vi "Waveform and Laser Controls V3.vi"() -> ()   [LabVIEW 2014]
uses:
  Waveform Scan Parameters.ctl
  <vilib>/Platform/TimedLoop/XDataNode/timing_clust.ctl
  <vilib>/Platform/TimedLoop/XDataNode/nitl_modes.ctl
  <vilib>/Platform/TimedLoop/XDataNode/wakeup.ctl
  <vilib>/rvi/Emulation/niFpgaGetClockAttributes.vi
  <vilib>/rvi/Emulation/niFpgaSctlEmulationGetInTimedLoop.vi
  <vilib>/rvi/Emulation/niFpgaEmulationReportErrorSimple.vi
  <vilib>/rvi/eio/common/nirviEmuTemplateMethod_errors.vi
  <vilib>/rvi/Emulation/niFpgaCriticalErrorInLSC.vi
  <vilib>/rvi/Memory/Memory_Emulation/nirvimemoryFastEmulation.vi
  <vilib>/rvi/Memory/Memory_Emulation/nirvimemoryEmulation.vi
  <vilib>/rvi/Emulation/niFpgaEmulationIsFPGAContextNoSignature.vi
  <vilib>/rvi/DataTransferAndStorage/Container/Common/niFpgaContainerGetUniqueNameForEmu.vi
  <vilib>/rvi/Emulation/niFpgaProcessEmulError.vi
  <vilib>/rvi/errors/nirviReportUnexpectedCaseInternalError (U32).vi
  <vilib>/eio/EIONode/EIONode.xnode
  <vilib>/rvi/DataTransferAndStorage/Container/XNode/niFpgaContainer.xnode
  <vilib>/Platform/TimedLoop/XDataNode/XDataNode.xnode
  <vilib>/Platform/TimedLoop/XDataNode/XDNodeRunTimeDep.lvlib
panel:
  out "End Linear Ramp":bool
  in  "End of Linear Ramp":u32
  in  "Z Stack Start Position (I16)":i16
  in  "Frames Per Z Step":u8
  in  "Number of Z Steps":u8
  in  "Z Step Size (I16)":i16
  in  "Stop Sync Signal":bool
  in  "Accums Per Line":u32[](array[numeric])=[0, 0, 0, 0]
  in  "Number of Lines":u32
  out "Frame Trigger":bool
  in  "Reset Position Error":bool
  in  "Galvo 1 Position (I16)":i16
  in  "Galvo 2 Position (I16)":i16
  in  "WF 3 Data Loaded":bool
  in  "WF 2 Data Loaded":bool
  in  "Waveform Scan Parameters":T1={"Scanning Mode"=0, "Fast Axis WF Length (Elements)"=0, "Fast Axis Sample Period (Ticks)"=40, "Slow Axis 1 WF Length (Elements)"=0, "Slow Axis 1 Sample Period (Ticks)"=40, "Slow Axis 1 Delay (25 ns) Steps"=40, "Slow Axis 2 WFLength (Elements)"=0, "Slow Axis 2 Sample Period (Ticks)"=40, "Slow Axis 2 Delay (25 ns) Steps"=40}
  in  "Resonant Mirror":T2
  in  "775 AOM":T3={"AOM (Pin 51 AO4)"=16500, "Beam Blanking"=FALSE}
  in  "Galvo Mirror 2":T4
  in  "Galvo Mirror 1":T4
  in  "Start Waveforms":bool
  in  "Unused Axis Offset":i16
  in  "Slow Axis 2 Waveform Element":i16
  in  "Fast Axis Waveform Element":i16
  in  "Slow Axis 1 Waveform Element":i16
  in  "WF 1 Data Loaded":bool
  # "V2 - Adding in a line clock\nV3 - Cluster Scan Parameters"
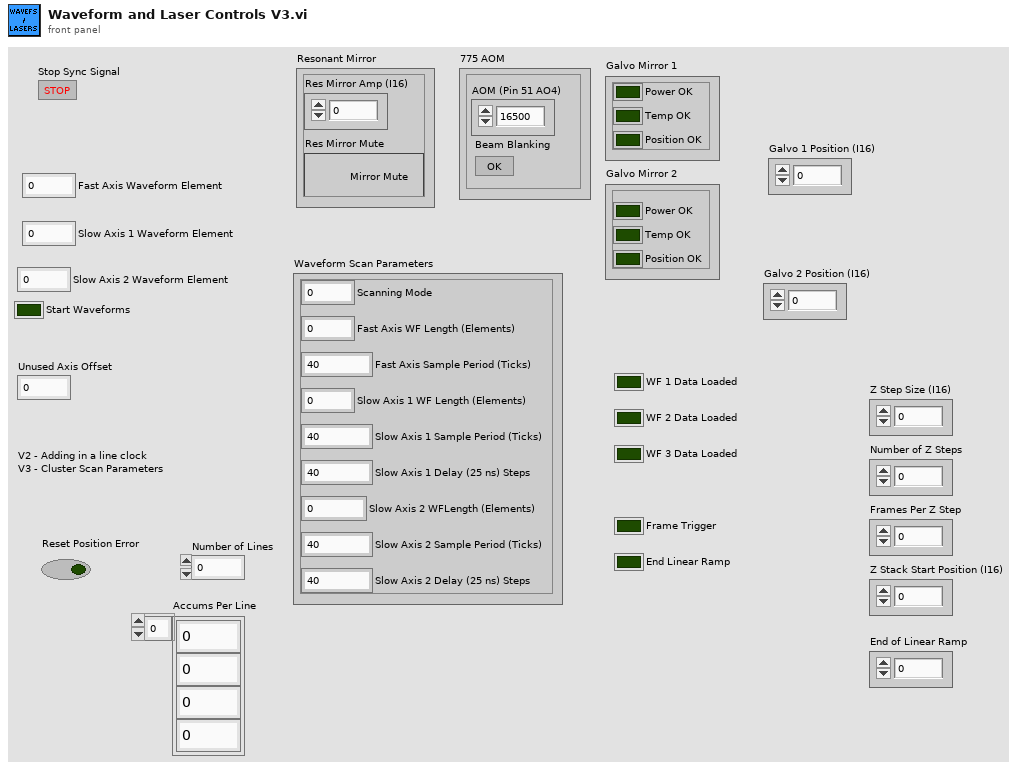
[diagram p1: front panel]
types:
  T1 = typedef "Waveform Scan Parameters.ctl" = cluster{"Scanning Mode":u8, "Fast Axis WF Length (Elements)":i32, "Fast Axis Sample Period (Ticks)":u32, "Slow Axis 1 WF Length (Elements)":i32, "Slow Axis 1 Sample Period (Ticks)":u32, "Slow Axis 1 Delay (25 ns) Steps":i32, "Slow Axis 2 WFLength (Elements)":i32, "Slow Axis 2 Sample Period (Ticks)":u32, "Slow Axis 2 Delay (25 ns) Steps":i32}
  T2 = cluster{"Res Mirror Amp (I16)":i16, "Res Mirror Mute":bool}
  T3 = cluster{"AOM (Pin 51 AO4)":i16, "Beam Blanking":bool}
  T4 = cluster{"Power OK":bool, "Temp OK":bool, "Position OK":bool}
  T5 = typedef "XDNodeRunTimeDep.lvlib/timing_clust.ctl" = cluster{"Expected End [f-1]":u64, "Actual End [f-1]":u64, "Finished Late? [f-1]":bool, "Expected End [i-1]":u64, "Actual End [i-1]":u64, "Finished Late? [i-1]":bool, "Expected Start [i]":u64, "Actual Start [i]":u64, "Expected Start [f]":u64, "Actual Start [f]":u64, "Source Name":string, "Structure Name":string, "Period":i64, "Deadline":i64, "Offset":i64, "Start":i64, "Priority":i32, "Timeout":i32, "Mode":T6, "Wakeup Reason":T7, "Error":errorcluster, "Source Type":string, "Secondary Source Type":string, "Global End Time":u64, "Global Start Time":u64, "Frame Duration":u64, "Iteration Duration":u64, "Assigned CPU":i32, "I/O Scan Engine Mode":u32}
  T6 = typedef "XDNodeRunTimeDep.lvlib/nitl_modes.ctl" = enum32{"No Change", "Process missed periods, maintain original phase", "Discard missed periods, maintain original phase", "Process missed periods, ignore original phase", "Discard missed periods, ignore original phase"}
  T7 = typedef "XDNodeRunTimeDep.lvlib/wakeup.ctl" = enum32{"Normal", "Aborted", "Asynchronous wakeup", "Timing source error", "Timed loop error", "Timeout"}
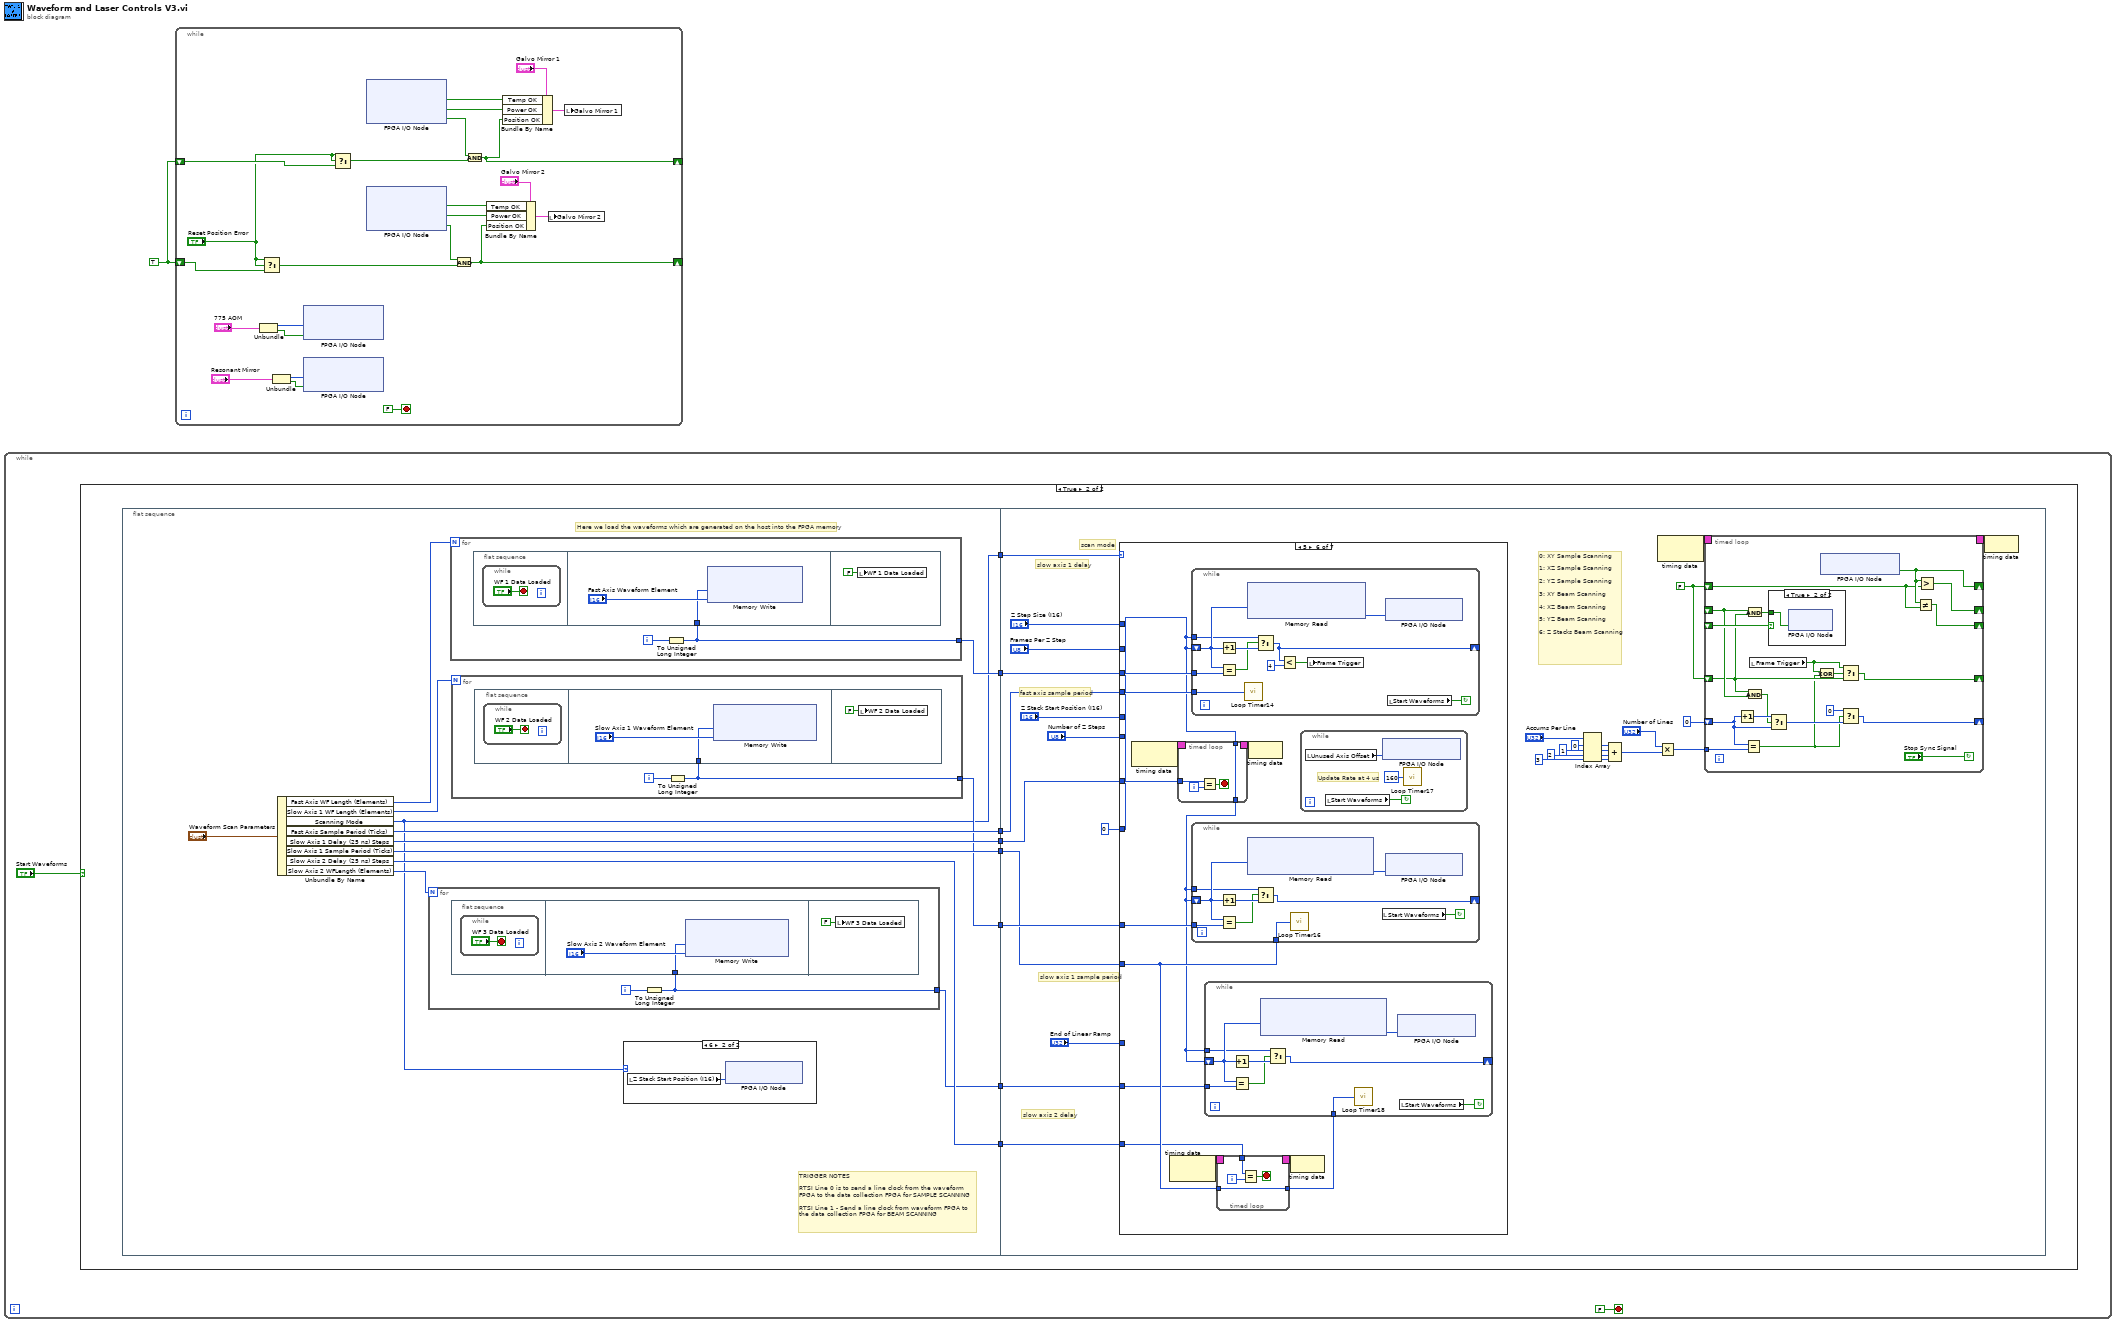
[diagram p0: block diagram]
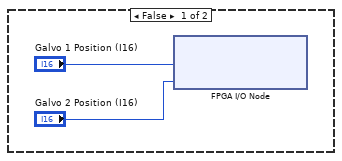
[diagram p2: hidden frame]
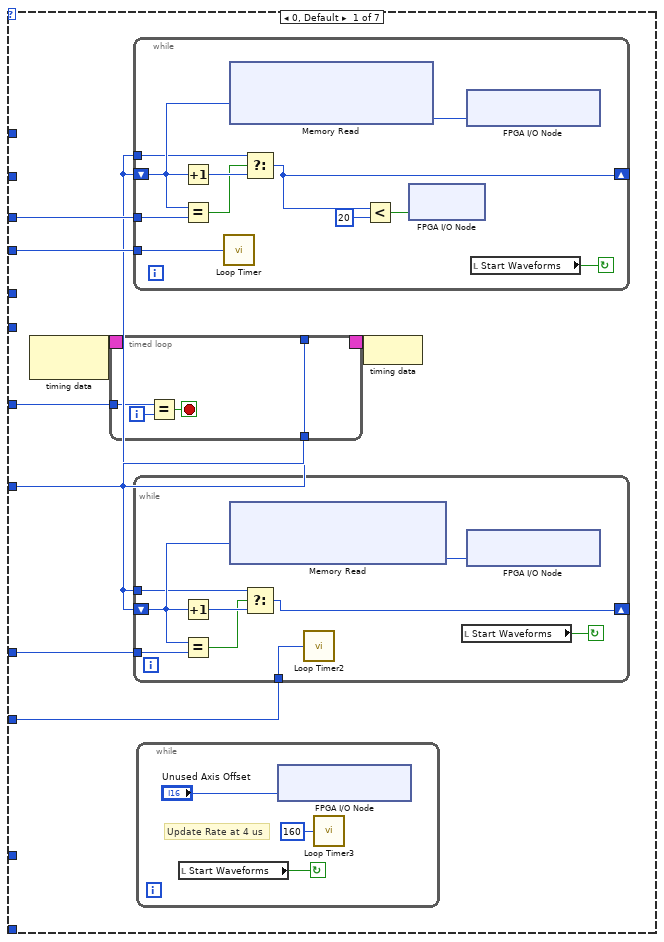
[diagram p5: hidden frame]
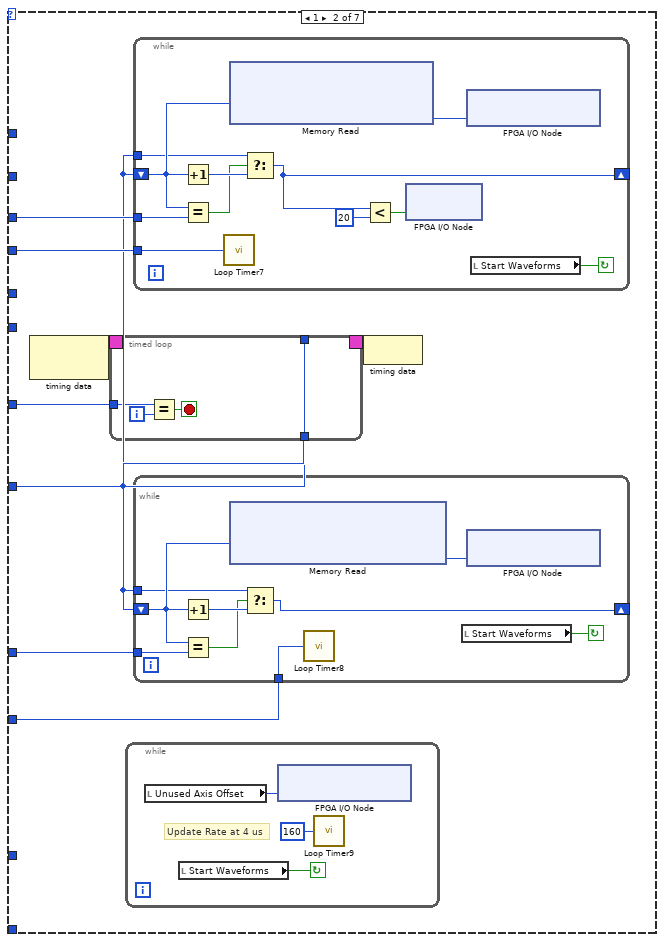
[diagram p6: hidden frame]
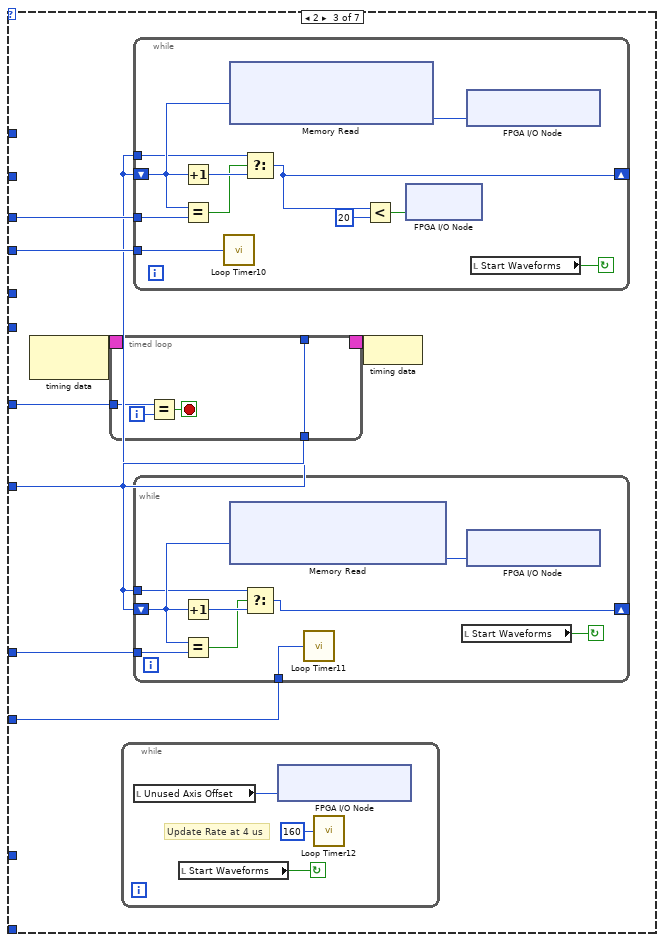
[diagram p7: hidden frame]
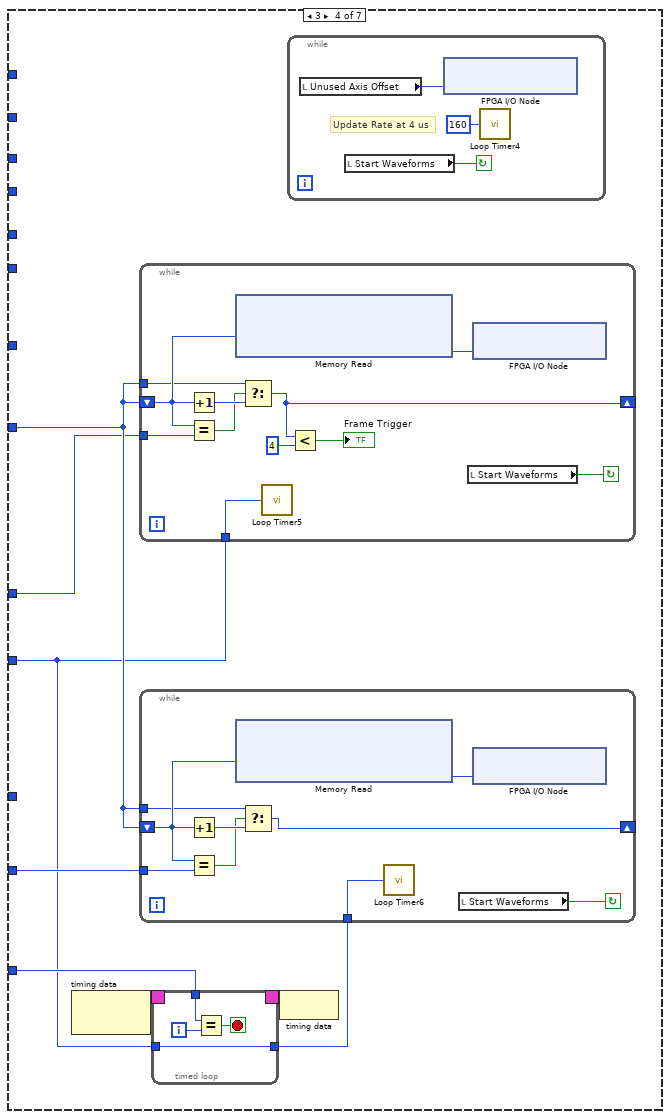
[diagram p8: hidden frame]
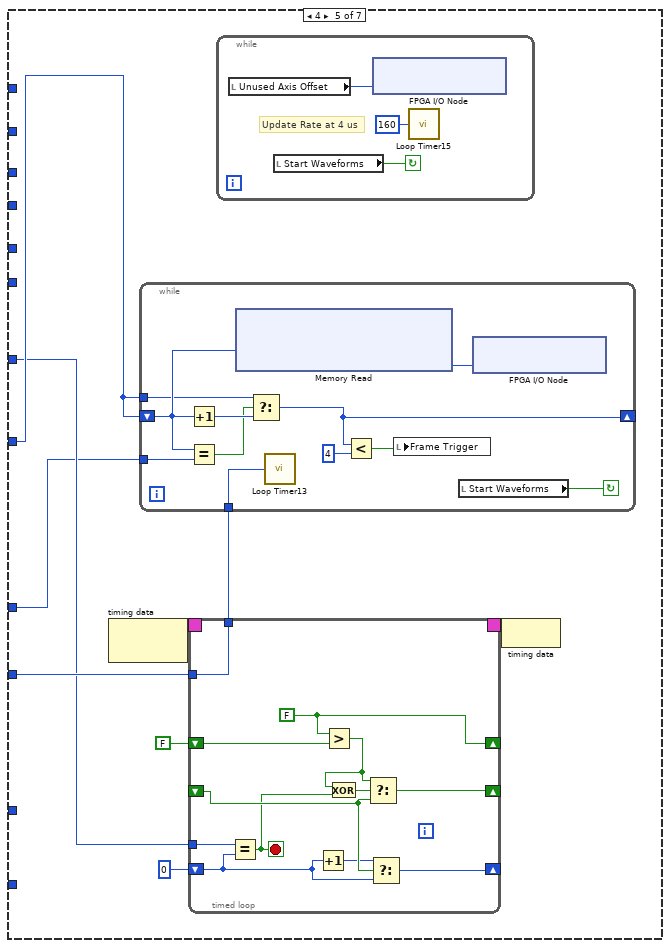
[diagram p9: hidden frame]
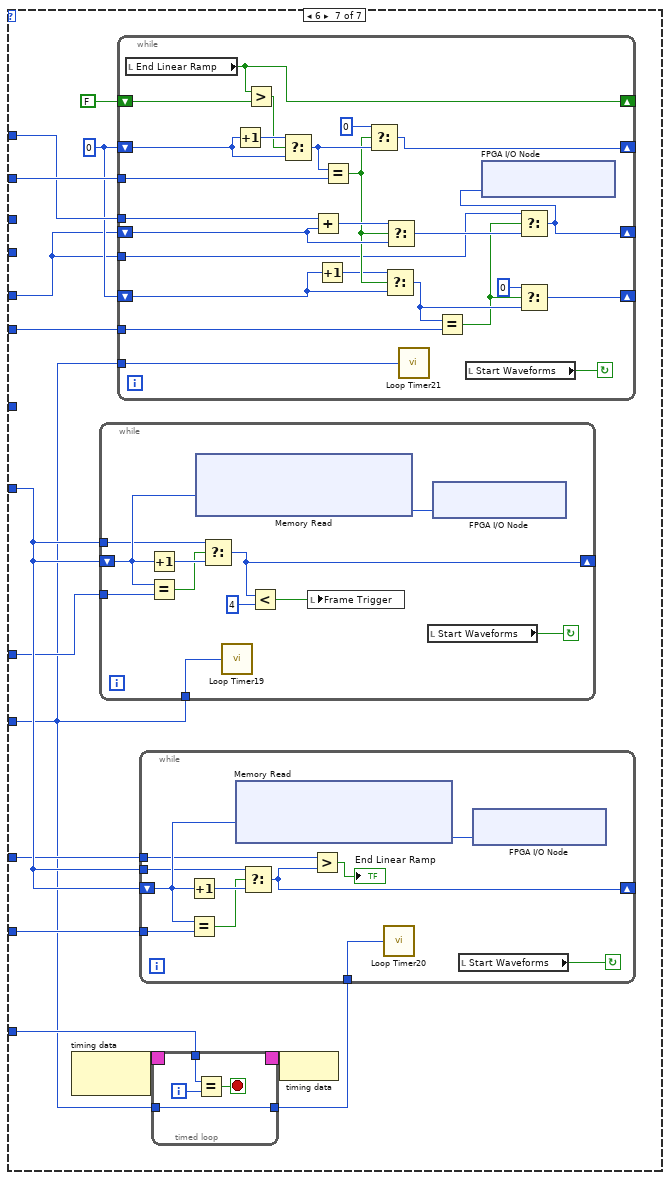
[diagram p10: hidden frame]
diagram:
  w1 = TRUE
  n1 = while {
    stop <- FALSE stop-if-true
    n2 = case shown="True" "Start Waveforms" {
      frame False {
        n3 = xnode "FPGA I/O Node"("Connector0/AO5"="Galvo 1 Position (I16)", "Connector0/AO6"="Galvo 2 Position (I16)") -> ()  [unwired: 2 in, 2 out]
      }
      frame True {
        n4 = flat-sequence {
          tunnel: [w25] -> w13
          tunnel: [w15] -> w12
          tunnel: [w16] -> w11
          tunnel: [w14] -> w10
          tunnel: [w23] -> w9
          tunnel: [w22] -> w8
          tunnel: [w21] -> w7
          tunnel: [w20] -> w6
          tunnel: w13 -> [w74]
          tunnel: w12 -> [w73]
          tunnel: w11 -> [w71]
          tunnel: w10 -> [w70]
          tunnel: w9 -> [w69]
          tunnel: w8 -> [w68]
          tunnel: w7 -> [w67]
          tunnel: w6 -> [w66]
          frame #0 {
            # "TRIGGER NOTES\n\nRTSI Line 0 is to send a line clock from the waveform\nFPGA to the data collection FPGA for SAMPLE SCANNING\n\nRTSI Line 1 - Send a line clock from waveform FPGA to\nthe data collection FPGA for BEAM SCANNING"
            # "Here we load the waveforms which are generated on the host into the FPGA memory"
            n5 = Unbundle By Name("Waveform Scan Parameters") -> ("Fast Axis WF Length (Elements)"=w19:i32, "Slow Axis 1 WF Length (Elements)"=w18:i32, "Scanning Mode"=w14:u8, "Fast Axis Sample Period (Ticks)"=w23:u32, "Slow Axis 1 Delay (25 ns) Steps"=w22:i32, "Slow Axis 1 Sample Period (Ticks)"=w21:u32, "Slow Axis 2 Delay (25 ns) Steps"=w20:i32, "Slow Axis 2 WFLength (Elements)"=w17:i32)
            n6 = for {
              N: w17 -> [_]
              tunnel: [w27] -> w15
              i -> [w28]
              n7 = flat-sequence {
                tunnel: w27 -> [w30]
                frame #0 {
                  n8 = while {
                    stop <- "WF 3 Data Loaded" stop-if-true
                  }
                }
                frame #1 {
                  n9 = xnode ("Memory Write")("Address"=w30, "Data"="Slow Axis 2 Waveform Element") -> ()  [unwired: 1 in, 1 out]
                }
                frame #2 {
                  n10 = local write "WF 3 Data Loaded"(FALSE ("Host Data Loaded")) -> ()
                }
              }
              n11 = To Unsigned Long Integer(number=w28) -> (unsigned 32bit integer=w27:u32)
            }
            n12 = for {
              N: w19 -> [_]
              tunnel: [w39] -> w25
              i -> [w40]
              n13 = flat-sequence {
                tunnel: w39 -> [w42]
                frame #0 {
                  n14 = while {
                    stop <- "WF 1 Data Loaded" stop-if-true
                  }
                }
                frame #1 {
                  n15 = xnode ("Memory Write")("Address"=w42, "Data"="Fast Axis Waveform Element") -> ()  [unwired: 1 in, 1 out]
                }
                frame #2 {
                  n16 = local write "WF 1 Data Loaded"(FALSE ("Host Data Loaded")) -> ()
                }
              }
              n17 = To Unsigned Long Integer(number=w40) -> (unsigned 32bit integer=w39:u32)
            }
            n18 = for {
              N: w18 -> [_]
              tunnel: [w33] -> w16
              i -> [w34]
              n19 = flat-sequence {
                tunnel: w33 -> [w36]
                frame #0 {
                  n20 = while {
                    stop <- "WF 2 Data Loaded" stop-if-true
                  }
                }
                frame #1 {
                  n21 = xnode ("Memory Write")("Address"=w36, "Data"="Slow Axis 1 Waveform Element") -> ()  [unwired: 1 in, 1 out]
                }
                frame #2 {
                  n22 = local write "WF 2 Data Loaded"(FALSE ("Host Data Loaded")) -> ()
                }
              }
              n23 = To Unsigned Long Integer(number=w34) -> (unsigned 32bit integer=w33:u32)
            }
            n24 = case shown="6" w14 {
              frame 0, Default {
              }
              frame 6 {
                n25 = local read "Z Stack Start Position (I16)"() -> (w26:i16)
                n26 = xnode "FPGA I/O Node"("Connector0/AO3"=w26) -> ()  [unwired: 1 in, 1 out]
              }
            }
          }
          frame #1 {
            w51 = FALSE
            # "slow axis 2 delay"
            # "slow axis 1 sample period"
            # "slow axis 1 delay"
            # "fast axis sample period"
            # "scan mode"
            # "0: XY Sample Scanning\n\n1: XZ Sample Scanning\n\n2: YZ Sample Scanning\n\n3: XY Beam Scanning\n\n4: XZ Beam Scanning\n\n5: YZ Beam Scanning\n\n6: Z Stacks Beam Scanning"
            n27 = case shown="5" w70 {
              tunnel: w74 -> [w106 w146 w186 _ _ w311 _]
              tunnel: w69 -> [w105 w145 w185 _ _ w310 _]
              tunnel: w73 -> [_ _ _ w227 _ w305 w374]
              tunnel: u32 0 -> [w100 w140 w180 w226 w267 w307 w373]
              tunnel: w68 -> [w104 w144 w184 _ w265 w309 _]
              tunnel: w66 -> [_ _ _ w225 _ w304 w372]
              tunnel: w71 -> [w102 w142 w182 w220 w264 w308 w369]
              tunnel: w67 -> [w101 w141 w181 w221 w266 w306 w360]
              tunnel: "Frames Per Z Step" -> [_ _ _ _ _ _ w367]
              tunnel: "Z Stack Start Position (I16)" -> [_ _ _ _ _ _ w363]
              tunnel: "Z Step Size (I16)" -> [_ _ _ _ _ _ w366]
              tunnel: "Number of Z Steps" -> [_ _ _ _ _ _ w364]
              tunnel: "End of Linear Ramp" -> [_ _ _ _ _ _ w362]
              frame 0, Default {
                n28 = node-c288() -> (w108:T5)  [unwired: 1 in]
                n29 = timed-loop {
                  timing: w108 -> [_]
                  timing-out: [_] -> w107
                  tunnel: w104 -> [w113]
                  tunnel: w100 -> [w112]
                  tunnel: [w112] -> w103
                  i -> [w115]
                  stop <- w114 stop-if-true
                  n30 = Equal?(x=w113, y=w115) -> (x = y?=w114:bool)
                }
                n31 = while {
                  shift-right: [w131] -> _
                  shift-left: w100 -> [w137]
                  tunnel: w106 -> [w138]
                  tunnel: w105 -> [w135]
                  tunnel: w100 -> [w134]
                  stop <- w133 continue-if-true
                  n32 = Increment(x=w137) -> (x+1=w139:u32)
                  n33 = Equal?(x=w137, y=w138) -> (x = y?=w132:bool)
                  n34 = call "Loop Timer"("Count(Ticks)"=w135) -> ()  [unwired: 1 out]
                  n35 = xnode ("Memory Read")("Address"=w137) -> ("Data"=w136:i16)  [unwired: 1 in, 1 out]
                  n36 = Select(t=w134, s=w132, f=w139) -> (s? t:f=w131:u32)
                  n37 = Less?(x=w131, y=u32 20) -> (x < y?=w129:bool)
                  n38 = xnode "FPGA I/O Node"("TRIG0"=w129) -> ()  [unwired: 1 in, 1 out]
                  n39 = xnode "FPGA I/O Node"("Connector0/AO1"=w136) -> ()  [unwired: 1 in, 1 out]
                  n40 = local read "Start Waveforms"() -> (w133:bool)
                }
                n41 = while {
                  shift-right: [w127] -> _
                  shift-left: w103 -> [w124]
                  tunnel: w102 -> [w126]
                  tunnel: w103 -> [w122]
                  tunnel: w101 -> [w121]
                  stop <- w120 continue-if-true
                  n42 = Increment(x=w124) -> (x+1=w128:u32)
                  n43 = Equal?(x=w124, y=w126) -> (x = y?=w125:bool)
                  n44 = xnode ("Memory Read")("Address"=w124) -> ("Data"=w123:i16)  [unwired: 1 in, 1 out]
                  n45 = Select(t=w122, s=w125, f=w128) -> (s? t:f=w127:u32)
                  n46 = call "Loop Timer2"("Count(Ticks)"=w121) -> ()  [unwired: 1 out]
                  n47 = local read "Start Waveforms"() -> (w120:bool)
                  n48 = xnode "FPGA I/O Node"("Connector0/AO2"=w123) -> ()  [unwired: 1 in, 1 out]
                }
                n49 = while {
                  stop <- w109 continue-if-true
                  # "Update Rate at 4 us"
                  n50 = local read "Start Waveforms"() -> (w109:bool)
                  n51 = xnode "FPGA I/O Node"("Connector0/AO3"="Unused Axis Offset") -> ()  [unwired: 1 in, 1 out]
                  n52 = call "Loop Timer3"("Count(Ticks)"=u32 160) -> ()  [unwired: 1 out]
                }
                n53 = node-c288(w107) -> ()
              }
              frame 1 {
                n54 = node-c288() -> (w148:T5)  [unwired: 1 in]
                n55 = timed-loop {
                  timing: w148 -> [_]
                  timing-out: [_] -> w147
                  tunnel: w144 -> [w153]
                  tunnel: w140 -> [w152]
                  tunnel: [w152] -> w143
                  i -> [w155]
                  stop <- w154 stop-if-true
                  n56 = Equal?(x=w153, y=w155) -> (x = y?=w154:bool)
                }
                n57 = while {
                  stop <- w150 continue-if-true
                  # "Update Rate at 4 us"
                  n58 = local read "Unused Axis Offset"() -> (w149:i16)
                  n59 = local read "Start Waveforms"() -> (w150:bool)
                  n60 = xnode "FPGA I/O Node"("Connector0/AO2"=w149) -> ()  [unwired: 1 in, 1 out]
                  n61 = call "Loop Timer9"("Count(Ticks)"=u32 160) -> ()  [unwired: 1 out]
                }
                n62 = while {
                  shift-right: [w171] -> _
                  shift-left: w140 -> [w177]
                  tunnel: w146 -> [w178]
                  tunnel: w145 -> [w175]
                  tunnel: w140 -> [w174]
                  stop <- w173 continue-if-true
                  n63 = Increment(x=w177) -> (x+1=w179:u32)
                  n64 = Equal?(x=w177, y=w178) -> (x = y?=w172:bool)
                  n65 = call "Loop Timer7"("Count(Ticks)"=w175) -> ()  [unwired: 1 out]
                  n66 = xnode ("Memory Read")("Address"=w177) -> ("Data"=w176:i16)  [unwired: 1 in, 1 out]
                  n67 = Select(t=w174, s=w172, f=w179) -> (s? t:f=w171:u32)
                  n68 = Less?(x=w171, y=u32 20) -> (x < y?=w169:bool)
                  n69 = xnode "FPGA I/O Node"("TRIG0"=w169) -> ()  [unwired: 1 in, 1 out]
                  n70 = xnode "FPGA I/O Node"("Connector0/AO1"=w176) -> ()  [unwired: 1 in, 1 out]
                  n71 = local read "Start Waveforms"() -> (w173:bool)
                }
                n72 = while {
                  shift-right: [w167] -> _
                  shift-left: w143 -> [w164]
                  tunnel: w142 -> [w166]
                  tunnel: w143 -> [w162]
                  tunnel: w141 -> [w161]
                  stop <- w160 continue-if-true
                  n73 = Increment(x=w164) -> (x+1=w168:u32)
                  n74 = Equal?(x=w164, y=w166) -> (x = y?=w165:bool)
                  n75 = xnode ("Memory Read")("Address"=w164) -> ("Data"=w163:i16)  [unwired: 1 in, 1 out]
                  n76 = Select(t=w162, s=w165, f=w168) -> (s? t:f=w167:u32)
                  n77 = call "Loop Timer8"("Count(Ticks)"=w161) -> ()  [unwired: 1 out]
                  n78 = local read "Start Waveforms"() -> (w160:bool)
                  n79 = xnode "FPGA I/O Node"("Connector0/AO3"=w163) -> ()  [unwired: 1 in, 1 out]
                }
                n80 = node-c288(w147) -> ()
              }
              frame 2 {
                n81 = node-c288() -> (w188:T5)  [unwired: 1 in]
                n82 = timed-loop {
                  timing: w188 -> [_]
                  timing-out: [_] -> w187
                  tunnel: w184 -> [w193]
                  tunnel: w180 -> [w192]
                  tunnel: [w192] -> w183
                  i -> [w195]
                  stop <- w194 stop-if-true
                  n83 = Equal?(x=w193, y=w195) -> (x = y?=w194:bool)
                }
                n84 = while {
                  stop <- w190 continue-if-true
                  # "Update Rate at 4 us"
                  n85 = local read "Unused Axis Offset"() -> (w189:i16)
                  n86 = local read "Start Waveforms"() -> (w190:bool)
                  n87 = xnode "FPGA I/O Node"("Connector0/AO1"=w189) -> ()  [unwired: 1 in, 1 out]
                  n88 = call "Loop Timer12"("Count(Ticks)"=u32 160) -> ()  [unwired: 1 out]
                }
                n89 = while {
                  shift-right: [w211] -> _
                  shift-left: w180 -> [w217]
                  tunnel: w186 -> [w218]
                  tunnel: w185 -> [w215]
                  tunnel: w180 -> [w214]
                  stop <- w213 continue-if-true
                  n90 = Increment(x=w217) -> (x+1=w219:u32)
                  n91 = Equal?(x=w217, y=w218) -> (x = y?=w212:bool)
                  n92 = call "Loop Timer10"("Count(Ticks)"=w215) -> ()  [unwired: 1 out]
                  n93 = xnode ("Memory Read")("Address"=w217) -> ("Data"=w216:i16)  [unwired: 1 in, 1 out]
                  n94 = Select(t=w214, s=w212, f=w219) -> (s? t:f=w211:u32)
                  n95 = Less?(x=w211, y=u32 20) -> (x < y?=w209:bool)
                  n96 = xnode "FPGA I/O Node"("TRIG0"=w209) -> ()  [unwired: 1 in, 1 out]
                  n97 = xnode "FPGA I/O Node"("Connector0/AO2"=w216) -> ()  [unwired: 1 in, 1 out]
                  n98 = local read "Start Waveforms"() -> (w213:bool)
                }
                n99 = while {
                  shift-right: [w207] -> _
                  shift-left: w183 -> [w204]
                  tunnel: w182 -> [w206]
                  tunnel: w183 -> [w202]
                  tunnel: w181 -> [w201]
                  stop <- w200 continue-if-true
                  n100 = Increment(x=w204) -> (x+1=w208:u32)
                  n101 = Equal?(x=w204, y=w206) -> (x = y?=w205:bool)
                  n102 = xnode ("Memory Read")("Address"=w204) -> ("Data"=w203:i16)  [unwired: 1 in, 1 out]
                  n103 = Select(t=w202, s=w205, f=w208) -> (s? t:f=w207:u32)
                  n104 = call "Loop Timer11"("Count(Ticks)"=w201) -> ()  [unwired: 1 out]
                  n105 = local read "Start Waveforms"() -> (w200:bool)
                  n106 = xnode "FPGA I/O Node"("Connector0/AO3"=w203) -> ()  [unwired: 1 in, 1 out]
                }
                n107 = node-c288(w187) -> ()
              }
              frame 3 {
                n108 = node-c288() -> (w224:T5)  [unwired: 1 in]
                n109 = while {
                  shift-right: [w250] -> _
                  shift-left: w226 -> [w256]
                  tunnel: w220 -> [w257]
                  tunnel: w221 -> [w254]
                  tunnel: w226 -> [w253]
                  stop <- w252 continue-if-true
                  n110 = Increment(x=w256) -> (x+1=w258:u32)
                  n111 = Equal?(x=w256, y=w257) -> (x = y?=w251:bool)
                  n112 = xnode ("Memory Read")("Address"=w256) -> ("Data"=w255:i16)  [unwired: 1 in, 1 out]
                  n113 = Select(t=w253, s=w251, f=w258) -> (s? t:f=w250:u32)
                  n114 = call "Loop Timer5"("Count(Ticks)"=w254) -> ()  [unwired: 1 out]
                  n115 = Less?(x=w250, y=u32 4) -> (x < y?=→"Frame Trigger":bool)
                  n116 = local read "Start Waveforms"() -> (w252:bool)
                  n117 = xnode "FPGA I/O Node"("Connector0/AO5"=w255) -> ()  [unwired: 1 in, 1 out]
                }
                n118 = timed-loop {
                  timing: w224 -> [_]
                  timing-out: [_] -> w223
                  tunnel: w221 -> [w240]
                  tunnel: [w240] -> w222
                  tunnel: w225 -> [w241]
                  i -> [w243]
                  stop <- w242 stop-if-true
                  n119 = Equal?(x=w241, y=w243) -> (x = y?=w242:bool)
                }
                n120 = while {
                  shift-right: [w238] -> _
                  shift-left: w226 -> [w236]
                  tunnel: w227 -> [w237]
                  tunnel: w222 -> [w234]
                  tunnel: w226 -> [w233]
                  stop <- w232 continue-if-true
                  n121 = Increment(x=w236) -> (x+1=w239:u32)
                  n122 = Equal?(x=w236, y=w237) -> (x = y?=w231:bool)
                  n123 = xnode ("Memory Read")("Address"=w236) -> ("Data"=w235:i16)  [unwired: 1 in, 1 out]
                  n124 = Select(t=w233, s=w231, f=w239) -> (s? t:f=w238:u32)
                  n125 = call "Loop Timer6"("Count(Ticks)"=w234) -> ()  [unwired: 1 out]
                  n126 = local read "Start Waveforms"() -> (w232:bool)
                  n127 = xnode "FPGA I/O Node"("Connector0/AO6"=w235) -> ()  [unwired: 1 in, 1 out]
                }
                n128 = node-c288(w223) -> ()
                n129 = while {
                  stop <- w229 continue-if-true
                  # "Update Rate at 4 us"
                  n130 = local read "Unused Axis Offset"() -> (w228:i16)
                  n131 = local read "Start Waveforms"() -> (w229:bool)
                  n132 = xnode "FPGA I/O Node"("Connector0/AO3"=w228) -> ()  [unwired: 1 in, 1 out]
                  n133 = call "Loop Timer4"("Count(Ticks)"=u32 160) -> ()  [unwired: 1 out]
                }
              }
              frame 4 {
                n134 = node-c288() -> (w263:T5)  [unwired: 1 in]
                n135 = timed-loop {
                  timing: w263 -> [_]
                  timing-out: [_] -> w262
                  tunnel: w266 -> [w273]
                  shift-right: [w271] -> _
                  shift-left: FALSE -> [w282]
                  shift-right: [w279] -> _
                  shift-left: _ -> [w278]
                  shift-right: [w276] -> _
                  shift-left: 0 -> [w274]
                  tunnel: w265 -> [w275]
                  tunnel: [w273] -> w259
                  stop <- w272 stop-if-true
                  w271 = FALSE
                  n136 = Equal?(x=w275, y=w274) -> (x = y?=w272:bool)
                  n137 = Increment(x=w274) -> (x+1=w277:i32)
                  n138 = Greater?(x=w271, y=w282) -> (0:w280:bool)
                  n139 = Exclusive Or(1:w272, 2:w280) -> (0:w281:bool)
                  n140 = Select(t=w280, s=w281, f=w278) -> (s? t:f=w279:bool)
                  n141 = Select(t=w277, s=w278, f=w274) -> (s? t:f=w276:i32)
                }
                n142 = while {
                  shift-right: [w288] -> _
                  shift-left: w267 -> [w294]
                  tunnel: w264 -> [w296]
                  tunnel: w259 -> [w292]
                  tunnel: w267 -> [w291]
                  stop <- w290 continue-if-true
                  n143 = Increment(x=w294) -> (x+1=w297:u32)
                  n144 = Equal?(x=w294, y=w296) -> (x = y?=w295:bool)
                  n145 = xnode ("Memory Read")("Address"=w294) -> ("Data"=w293:i16)  [unwired: 1 in, 1 out]
                  n146 = Select(t=w291, s=w295, f=w297) -> (s? t:f=w288:u32)
                  n147 = call "Loop Timer13"("Count(Ticks)"=w292) -> ()  [unwired: 1 out]
                  n148 = Less?(x=w288, y=u32 4) -> (x < y?=w287:bool)
                  n149 = local write "Frame Trigger"(w287) -> ()
                  n150 = local read "Start Waveforms"() -> (w290:bool)
                  n151 = xnode "FPGA I/O Node"("Connector0/AO3"=w293) -> ()  [unwired: 1 in, 1 out]
                }
                n152 = while {
                  stop <- w269 continue-if-true
                  # "Update Rate at 4 us"
                  n153 = local read "Unused Axis Offset"() -> (w268:i16)
                  n154 = local read "Start Waveforms"() -> (w269:bool)
                  n155 = xnode "FPGA I/O Node"("Connector0/AO2"=w268) -> ()  [unwired: 1 in, 1 out]
                  n156 = call "Loop Timer15"("Count(Ticks)"=u32 160) -> ()  [unwired: 1 out]
                }
                n157 = node-c288(w262) -> ()
              }
              frame 5 {
                n158 = node-c288() -> (w303:T5)  [unwired: 1 in]
                n159 = node-c288() -> (w301:T5)  [unwired: 1 in]
                n160 = timed-loop {
                  timing: w303 -> [_]
                  timing-out: [_] -> w302
                  tunnel: w309 -> [w333]
                  tunnel: w307 -> [w332]
                  tunnel: [w332] -> w298
                  i -> [w335]
                  stop <- w334 stop-if-true
                  n161 = Equal?(x=w333, y=w335) -> (x = y?=w334:bool)
                }
                n162 = while {
                  shift-right: [w351] -> _
                  shift-left: w307 -> [w357]
                  tunnel: w311 -> [w358]
                  tunnel: w310 -> [w355]
                  tunnel: w307 -> [w354]
                  stop <- w353 continue-if-true
                  n163 = Increment(x=w357) -> (x+1=w359:u32)
                  n164 = Equal?(x=w357, y=w358) -> (x = y?=w352:bool)
                  n165 = call "Loop Timer14"("Count(Ticks)"=w355) -> ()  [unwired: 1 out]
                  n166 = xnode ("Memory Read")("Address"=w357) -> ("Data"=w356:i16)  [unwired: 1 in, 1 out]
                  n167 = Select(t=w354, s=w352, f=w359) -> (s? t:f=w351:u32)
                  n168 = Less?(x=w351, y=u32 4) -> (x < y?=w349:bool)
                  n169 = local write "Frame Trigger"(w349) -> ()
                  n170 = xnode "FPGA I/O Node"("Connector0/AO5"=w356) -> ()  [unwired: 1 in, 1 out]
                  n171 = local read "Start Waveforms"() -> (w353:bool)
                }
                n172 = while {
                  shift-right: [w347] -> _
                  shift-left: w298 -> [w344]
                  tunnel: w308 -> [w346]
                  tunnel: w298 -> [w342]
                  tunnel: w306 -> [w341]
                  stop <- w340 continue-if-true
                  n173 = Increment(x=w344) -> (x+1=w348:u32)
                  n174 = Equal?(x=w344, y=w346) -> (x = y?=w345:bool)
                  n175 = xnode ("Memory Read")("Address"=w344) -> ("Data"=w343:i16)  [unwired: 1 in, 1 out]
                  n176 = Select(t=w342, s=w345, f=w348) -> (s? t:f=w347:u32)
                  n177 = call "Loop Timer16"("Count(Ticks)"=w341) -> ()  [unwired: 1 out]
                  n178 = local read "Start Waveforms"() -> (w340:bool)
                  n179 = xnode "FPGA I/O Node"("Connector0/AO6"=w343) -> ()  [unwired: 1 in, 1 out]
                }
                n180 = timed-loop {
                  timing: w301 -> [_]
                  timing-out: [_] -> w300
                  tunnel: w306 -> [w324]
                  tunnel: [w324] -> w299
                  tunnel: w304 -> [w325]
                  i -> [w327]
                  stop <- w326 stop-if-true
                  n181 = Equal?(x=w325, y=w327) -> (x = y?=w326:bool)
                }
                n182 = while {
                  shift-right: [w322] -> _
                  shift-left: w298 -> [w319]
                  tunnel: w305 -> [w321]
                  tunnel: w299 -> [w317]
                  tunnel: w298 -> [w316]
                  stop <- w315 continue-if-true
                  n183 = Increment(x=w319) -> (x+1=w323:u32)
                  n184 = Equal?(x=w319, y=w321) -> (x = y?=w320:bool)
                  n185 = xnode ("Memory Read")("Address"=w319) -> ("Data"=w318:i16)  [unwired: 1 in, 1 out]
                  n186 = Select(t=w316, s=w320, f=w323) -> (s? t:f=w322:u32)
                  n187 = call "Loop Timer18"("Count(Ticks)"=w317) -> ()  [unwired: 1 out]
                  n188 = xnode "FPGA I/O Node"("Connector0/AO3"=w318) -> ()  [unwired: 1 in, 1 out]
                  n189 = local read "Start Waveforms"() -> (w315:bool)
                }
                n190 = node-c288(w302) -> ()
                n191 = node-c288(w300) -> ()
                n192 = while {
                  stop <- w313 continue-if-true
                  # "Update Rate at 4 us"
                  n193 = local read "Unused Axis Offset"() -> (w312:i16)
                  n194 = local read "Start Waveforms"() -> (w313:bool)
                  n195 = xnode "FPGA I/O Node"("Connector0/AO1"=w312) -> ()  [unwired: 1 in, 1 out]
                  n196 = call "Loop Timer17"("Count(Ticks)"=u32 160) -> ()  [unwired: 1 out]
                }
              }
              frame 6 {
                w365 = u8 0
                n197 = node-c288() -> (w371:T5)  [unwired: 1 in]
                n198 = while {
                  shift-right: [w421] -> _
                  shift-left: w373 -> [w427]
                  tunnel: w369 -> [w428]
                  tunnel: w360 -> [w425]
                  tunnel: w373 -> [w424]
                  stop <- w423 continue-if-true
                  n199 = Increment(x=w427) -> (x+1=w429:u32)
                  n200 = Equal?(x=w427, y=w428) -> (x = y?=w422:bool)
                  n201 = xnode ("Memory Read")("Address"=w427) -> ("Data"=w426:i16)  [unwired: 1 in, 1 out]
                  n202 = Select(t=w424, s=w422, f=w429) -> (s? t:f=w421:u32)
                  n203 = call "Loop Timer19"("Count(Ticks)"=w425) -> ()  [unwired: 1 out]
                  n204 = Less?(x=w421, y=u32 4) -> (x < y?=w419:bool)
                  n205 = local write "Frame Trigger"(w419) -> ()
                  n206 = local read "Start Waveforms"() -> (w423:bool)
                  n207 = xnode "FPGA I/O Node"("Connector0/AO5"=w426) -> ()  [unwired: 1 in, 1 out]
                }
                n208 = while {
                  shift-right: [w397] -> _
                  shift-left: FALSE -> [w398]
                  shift-right: [w391] -> _
                  shift-left: w365 -> [w393]
                  tunnel: w367 -> [w392]
                  shift-right: [w375] -> _
                  shift-left: w363 -> [w388]
                  tunnel: w366 -> [w387]
                  shift-right: [w381] -> _
                  shift-left: w365 -> [w384]
                  tunnel: w364 -> [w380]
                  tunnel: w363 -> [w377]
                  tunnel: w360 -> [w376]
                  stop <- w399 continue-if-true
                  n209 = local read "End Linear Ramp"() -> (w397:bool)
                  n210 = Increment(x=w393) -> (x+1=w396:u8)
                  n211 = Greater?(x=w397, y=w398) -> (0:w395:bool)
                  n212 = Select(t=w396, s=w395, f=w393) -> (s? t:f=w390:u8)
                  n213 = Add(x=w387, y=w388) -> (x+y=w389:i16)
                  n214 = Increment(x=w384) -> (x+1=w385:u8)
                  n215 = Equal?(x=w390, y=w392) -> (x = y?=w386:bool)
                  n216 = Select(t=u8 0, s=w386, f=w390) -> (s? t:f=w391:u8)
                  n217 = Select(t=w385, s=w386, f=w384) -> (s? t:f=w382:u8)
                  n218 = Select(t=w389, s=w386, f=w388) -> (s? t:f=w383:i16)
                  n219 = call "Loop Timer21"("Count(Ticks)"=w376) -> ()  [unwired: 1 out]
                  n220 = Equal?(x=w382, y=w380) -> (x = y?=w379:bool)
                  n221 = local read "Start Waveforms"() -> (w399:bool)
                  n222 = Select(t=w377, s=w379, f=w383) -> (s? t:f=w375:i16)
                  n223 = xnode "FPGA I/O Node"("Connector0/AO3"=w375) -> ()  [unwired: 1 in, 1 out]
                  n224 = Select(t=u8 0, s=w379, f=w382) -> (s? t:f=w381:u8)
                }
                n225 = timed-loop {
                  timing: w371 -> [_]
                  timing-out: [_] -> w370
                  tunnel: w360 -> [w411]
                  tunnel: [w411] -> w361
                  tunnel: w372 -> [w412]
                  i -> [w414]
                  stop <- w413 stop-if-true
                  n226 = Equal?(x=w412, y=w414) -> (x = y?=w413:bool)
                }
                n227 = while {
                  shift-right: [w402] -> _
                  shift-left: w373 -> [w408]
                  tunnel: w374 -> [w409]
                  tunnel: w361 -> [w406]
                  tunnel: w373 -> [w405]
                  tunnel: w362 -> [w401]
                  stop <- w404 continue-if-true
                  n228 = Increment(x=w408) -> (x+1=w410:u32)
                  n229 = Equal?(x=w408, y=w409) -> (x = y?=w403:bool)
                  n230 = xnode ("Memory Read")("Address"=w408) -> ("Data"=w407:i16)  [unwired: 1 in, 1 out]
                  n231 = Select(t=w405, s=w403, f=w410) -> (s? t:f=w402:u32)
                  n232 = Greater?(x=w401, y=w402) -> (0:→"End Linear Ramp":bool)
                  n233 = call "Loop Timer20"("Count(Ticks)"=w406) -> ()  [unwired: 1 out]
                  n234 = local read "Start Waveforms"() -> (w404:bool)
                  n235 = xnode "FPGA I/O Node"("Connector0/AO6"=w407) -> ()  [unwired: 1 in, 1 out]
                }
                n236 = node-c288(w370) -> ()
              }
            }
            n237 = Index Array(array="Accums Per Line", index #1=0 ("index"), index #2=1 ("index"), index #3=2 ("index"), index #4=3 ("index")) -> (element #1=w55:u32, element #2=w54:u32, element #3=w53:u32, element #4=w52:u32)
            n238 = Compound Arithmetic op=ADD(w55, w54, w53, w52) -> (w62:u32)
            n239 = node-c288() -> (w65:T5)  [unwired: 1 in]
            n240 = Multiply(x="Number of Lines", y=w62) -> (x*y=w63:u32)
            n241 = timed-loop {
              timing: w65 -> [_]
              timing-out: [_] -> w64
              shift-right: [w94] -> _
              shift-left: w51 -> [w93]
              shift-right: [w91] -> _
              shift-left: _ -> [w84]
              shift-right: [w92] -> _
              shift-left: _ -> [w90]
              shift-right: [w76] -> _
              shift-left: u32 0 -> [w81]
              shift-right: [w86] -> _
              shift-left: w51 -> [w83]
              tunnel: w63 -> [w80]
              stop <- "Stop Sync Signal" continue-if-true
              n242 = Increment(x=w81) -> (x+1=w85:u32)
              n243 = Equal?(x=w81, y=w80) -> (x = y?=w78:bool)
              n244 = And(x=w84, y=w83) -> (x .and. y?=w89:bool)
              n245 = And(x=w83, y=w84) -> (x .and. y?=w82:bool)
              n246 = local read "Frame Trigger"() -> (w88:bool)
              n247 = case shown="True" w90 {
                tunnel: w89 -> [_ w95]
                frame False {
                }
                frame True {
                  n248 = xnode "FPGA I/O Node"("TRIG1"=w95) -> ()  [unwired: 1 in, 1 out]
                }
              }
              n249 = Select(t=w85, s=w82, f=w81) -> (s? t:f=w79:u32)
              n250 = Exclusive Or(1:w78, 2:w88) -> (0:w87:bool)
              n251 = xnode "FPGA I/O Node"() -> ("Connector1/DIO0"=w94:bool)  [unwired: 1 in, 1 out]
              n252 = Select(t=w88, s=w87, f=w83) -> (s? t:f=w86:bool)
              n253 = Select(t=u32 0, s=w78, f=w79) -> (s? t:f=w76:u32)
              n254 = Not Equal?(x=w94, y=w93) -> (x != y?=w92:bool)
              n255 = Greater?(x=w94, y=w93) -> (0:w91:bool)
            }
            n256 = node-c288(w64) -> ()
          }
        }
      }
    }
  }
  n257 = while {
    shift-right: [w435] -> _
    shift-left: w1 -> [w437]
    shift-right: [w431] -> _
    shift-left: w1 -> [w433]
    stop <- FALSE stop-if-true
    n258 = Unbundle("775 AOM") -> ("AOM (Pin 51 AO4)"=w451:i16, "Beam Blanking"=w450:bool)
    n259 = Select(t="Reset Position Error", s="Reset Position Error", f=w437) -> (s? t:f=w436:bool)
    n260 = Unbundle("Resonant Mirror") -> ("Res Mirror Amp (I16)"=w448:i16, "Res Mirror Mute"=w447:bool)
    n261 = xnode "FPGA I/O Node"("Connector0/AO4"=w451, "Connector0/DIO0"=w450) -> ()  [unwired: 3 in, 3 out]
    n262 = xnode "FPGA I/O Node"("Connector0/AO7"=w448, "Connector0/DIO7"=w447) -> ()  [unwired: 3 in, 3 out]
    n263 = Select(t="Reset Position Error", s="Reset Position Error", f=w433) -> (s? t:f=w432:bool)
    n264 = xnode "FPGA I/O Node"() -> ("Connector0/DIO1"=w446:bool, "Connector0/DIO2"=w445:bool, "Connector0/DIO3"=w434:bool)  [unwired: 4 in, 4 out]
    n265 = xnode "FPGA I/O Node"() -> ("Connector0/DIO4"=w439:bool, "Connector0/DIO5"=w440:bool, "Connector0/DIO6"=w438:bool)  [unwired: 4 in, 4 out]
    n266 = And(x=w438, y=w436) -> (x .and. y?=w435:bool)
    n267 = And(x=w434, y=w432) -> (x .and. y?=w431:bool)
    n268 = Bundle By Name(cluster="Galvo Mirror 2", "Temp OK"=w439, "Power OK"=w440, "Position OK"=w435) -> (w442:T4)
    n269 = Bundle By Name(cluster="Galvo Mirror 1", "Temp OK"=w446, "Power OK"=w445, "Position OK"=w431) -> (w444:T4)
    n270 = local write "Galvo Mirror 2"(w442) -> ()
    n271 = local write "Galvo Mirror 1"(w444) -> ()
  }
